vi "set_traces.vi"(8 "error in (no error)":errorcluster, 10 "traces (indices: ROI, sample)":sgl[][](array[numeric]), 11 "DL090623TwoDAnalyser.lvclass in":refnum<class "AnalyserDL090623TwoD.lvclass">) -> (0 "error out":errorcluster, 3 "DL090623TwoDAnalyser.lvclass out":refnum<class "AnalyserDL090623TwoD.lvclass">)   [LabVIEW 2010, in "AnalyserDL090623TwoD.lvclass"]
uses:
  AnalyserDL090623TwoD.lvclass
  AnalyserDL090623TwoD.lvclass/AnalyserDL090623TwoD.ctl
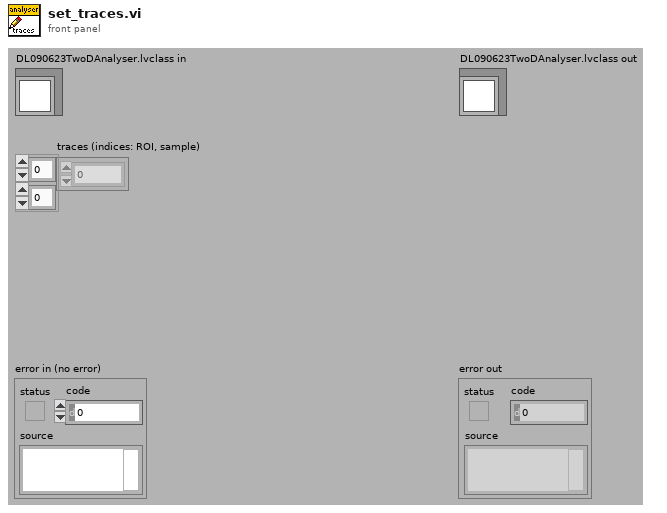
[diagram p1: front panel]
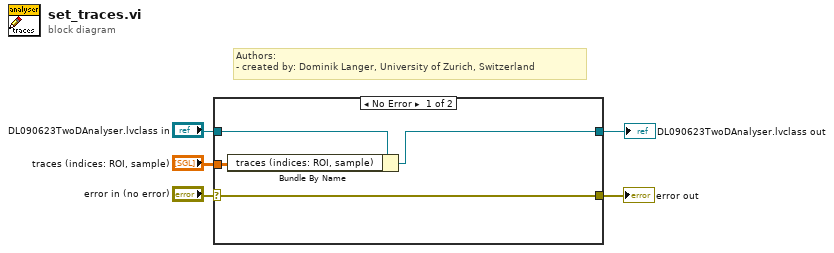
[diagram p0: block diagram]
diagram:
  # "Authors: \n- created by: Dominik Langer, University of Zurich, Switzerland"
  n1 = case shown="No Error" "error in (no error)" {
    selector: "error in (no error)" -> [w6 w10]
    tunnel: [w6 w10] -> w4
    tunnel: [w8 w11] -> w2
    tunnel: "DL090623TwoDAnalyser.lvclass in" -> [w9 w11]
    tunnel: "traces (indices: ROI, sample)" -> [w7 _]
    frame No Error {
      n2 = Bundle By Name(cluster=w9, "traces (indices: ROI, sample)"=w7) -> (w8:refnum<class "AnalyserDL090623TwoD.lvclass">)
    }
    frame Error {
    }
  }
  "error out" <- w4
  "DL090623TwoDAnalyser.lvclass out" <- w2
